vi "Set DDG Gate Time.vi"(10 "uiWidth":cluster{}, 11 "uiDelay":cluster{}) -> (3 "function return":u32)   [LabVIEW 2018, in "AndorSDK.lvlib"]
doc: "EXPNETTYPE unsigned int WINAPI SetDDGGateTime(at_u64 uiDelay, at_u64 uiWidth);"
uses:
  AndorSDK.lvlib
  ATMCD32D.dll
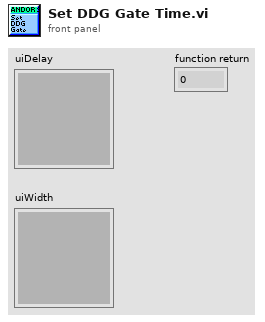
[diagram p1: front panel]
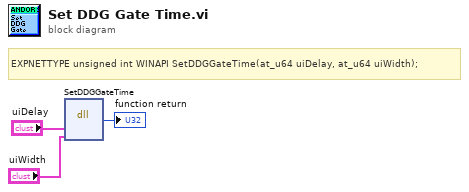
[diagram p0: block diagram]
diagram:
  # "EXPNETTYPE unsigned int WINAPI SetDDGGateTime(at_u64 uiDelay, at_u64 uiWidth);"
  n1 = dll-call lib="PTH2babs E\nPersönliches02 - Arbeit03-HiwijobsLabviewCodelibANDOR\tAndor SDK\nATMCD32D.*" fn="SetDDGGateTime"("uiDelay"="uiDelay", "uiWidth"="uiWidth") -> (→"function return":u32)  [unwired: 5 in, 2 out]
